vi "Scan DQMH Modules and create Maps.vi"(8 "error in":errorcluster, 10 "Include Dependencies":bool, 11 "Project":refnum<vi>) -> (0 "error out":errorcluster, 3 "DQMH Modules Info":T1)   [LabVIEW 2020, in "Dashboard.lvlib"]
doc: "Gets the Singleton and Cloneable references and creates a list of each type of DQMH Modules"
uses:
  Dashboard.lvlib
  DQMH Modules Info--cluster.ctl
  Module type--enum.ctl
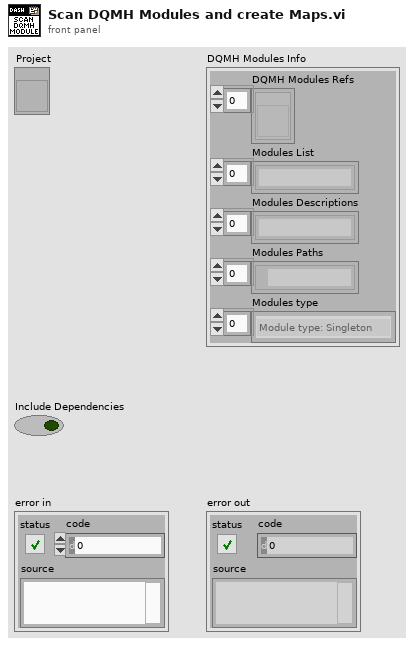
[diagram p1: front panel]
types:
  T1 = typedef "Dashboard.lvlib/DQMH Modules Info--cluster.ctl" = cluster{"DQMH Modules Refs":refnum<vi>[], "Modules List":string[], "Modules Descriptions":string[], "Modules Paths":path[], "Modules type":T2[]}
  T2 = typedef "Dashboard.lvlib/Module type--enum.ctl" = enum16{"Module type: Singleton", "Module type: Cloneable"}
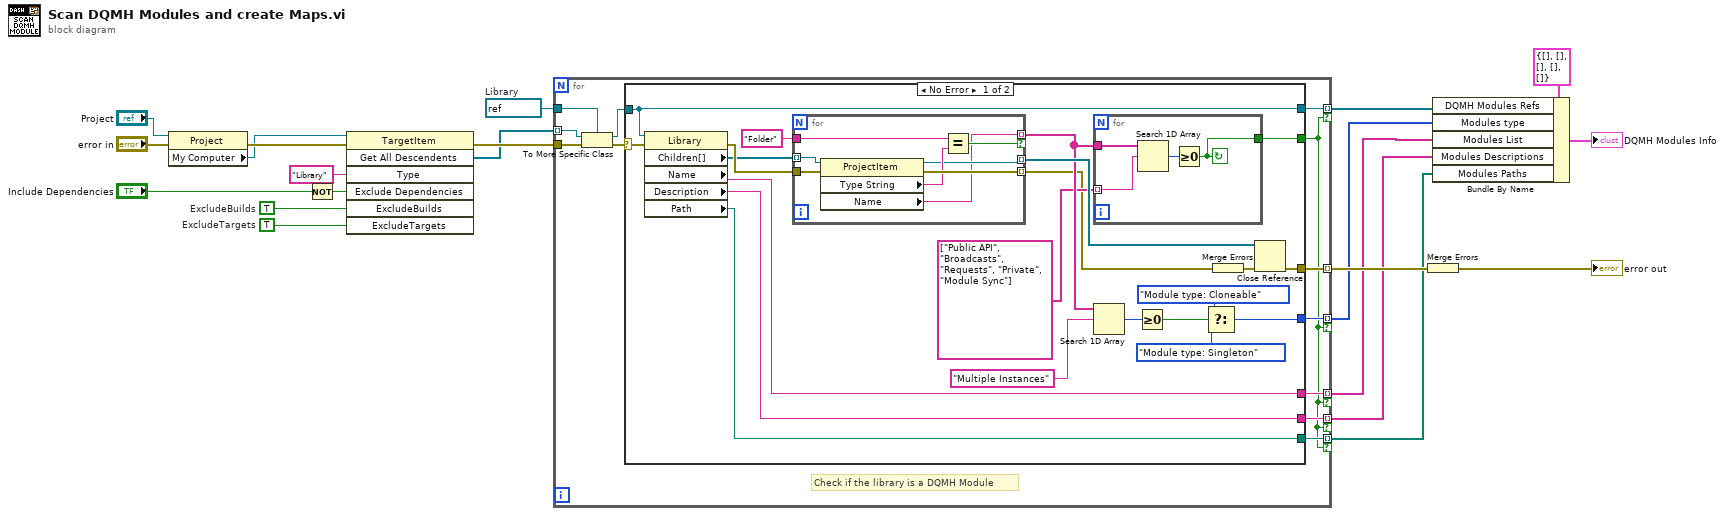
[diagram p0: block diagram]
diagram:
  w13 = refnum<vi> refnum  # Library
  w15 = TRUE  # ExcludeTargets
  w16 = TRUE  # ExcludeBuilds
  n1 = property class="Project"(reference="Project", error in="error in") -> (error out=w20:errorcluster, "My Computer"=w17:refnum<vi>)  [unwired: 1 out]
  n2 = Not(x="Include Dependencies") -> (.not. x?=w1:bool)
  n3 = invoke class="TargetItem" method="Get All Descendents"(reference=w17, error in=w20, "Type"="Library", "Exclude Dependencies"=w1, "ExcludeBuilds"=w16, "ExcludeTargets"=w15) -> (error out=w21:errorcluster, "All Descendents"=w12:refnum<vi>[])  [unwired: 1 in, 5 out]
  n4 = for {
    tunnel: w13 -> [w30]
    tunnel: [w29] -> w4 mode=indexing if=w22
    tunnel: w12 -> [w27] mode=indexing
    tunnel: [w32] -> w11 mode=indexing
    tunnel: w21 -> [w31]
    tunnel: [w26] -> w8 mode=indexing if=w22
    tunnel: [w25] -> w3 mode=indexing if=w22
    tunnel: [w24] -> w7 mode=indexing if=w22
    tunnel: [w23] -> w6 mode=indexing if=w22
    # "Check if the library is a DQMH Module"
    n5 = To More Specific Class(target class=w30, reference=w27, error in=w31) -> (specific class reference=w28:refnum<vi>, error out=w33:errorcluster)
    n6 = case shown="No Error" w33 {
      selector: w33 -> [w54 _]
      tunnel: w28 -> [w41 _]
      tunnel: [w50 _] -> w22
      tunnel: [w41 _] -> w29
      tunnel: [w53 _] -> w32
      tunnel: [w35 _] -> w26
      tunnel: [w40 _] -> w25
      tunnel: [w39 _] -> w24
      tunnel: [w38 _] -> w23
      frame No Error {
        n7 = property class="Library"(reference=w41, error in=w54) -> (error out=w52:errorcluster, "Children[]"=w48:refnum<vi>[], "Name"=w40:string, "Description"=w39:string, "Path"=w38:path)  [unwired: 1 out]
        n8 = for {
          tunnel: [w59] -> w44 mode=indexing if=w60
          tunnel: w52 -> [w66]
          tunnel: [w65] -> w42 mode=indexing
          tunnel: [w62] -> w47 mode=indexing
          tunnel: w48 -> [w64] mode=indexing
          tunnel: "Folder" ("Type") -> [w61]
          n9 = property class="ProjectItem"(reference=w64, error in=w66) -> (reference out=w62:refnum<vi>, error out=w65:errorcluster, "Type String"=w63:string, "Name"=w59:string)
          n10 = Equal?(x=w61, y=w63) -> (x = y?=w60:bool)
        }
        n11 = for {
          tunnel: string[] ["Public API", "Broadcasts", "Requests", "Private", "Module Sync"] -> [w58] mode=indexing
          tunnel: w44 -> [w57]
          tunnel: [w55] -> w50
          stop <- w55 continue-if-true
          n12 = Search 1D Array(1D array=w57, element=w58) -> (index of element=w56:i32)  [unwired: 1 in]
          n13 = Greater Or Equal To 0?(x=w56) -> (x >= 0?=w55:bool)
        }
        n14 = Search 1D Array(1D array=w44, element="Multiple Instances") -> (index of element=w46:i32)  [unwired: 1 in]
        n15 = Greater Or Equal To 0?(x=w46) -> (x >= 0?=w37:bool)
        n16 = Select(t=Module_type--enum."Module type: Cloneable", s=w37, f=Module_type--enum."Module type: Singleton" ("Module type")) -> (s? t:f=w35:T2)
        n17 = Merge Errors(w42) -> (w51:errorcluster)
        n18 = Close Reference(reference=w47, error in (no error)=w51) -> (error out=w53:errorcluster)
      }
      frame Error {
      }
    }
  }
  n19 = Merge Errors(w11) -> (→"error out":errorcluster)
  n20 = Bundle By Name(cluster=T1 {"DQMH Modules Refs"=[], "Modules List"=[], "Modules Descriptions"=[], "Modules Paths"=[], "Modules type"=[]} ("DQMH Modules Info"), "DQMH Modules Refs"=w4, "Modules type"=w8, "Modules List"=w3, "Modules Descriptions"=w7, "Modules Paths"=w6) -> (→"DQMH Modules Info":T1)
